vi "Measure distance.vi"(8 "error in (no error)":errorcluster, 11 "Input image":T3=refnum) -> (0 "error out":errorcluster)   [LabVIEW 2020]
uses:
  <vilib>/vision/Image Controls.llb/IMAQ Image.ctl
  <vilib>/vision/NI_Vision_Development_Module.lvlib
panel:
  in  "Clear Measurements":bool
  out "Distances":dbl[][](array[numeric])
  in  "Measurement Mode":T1(ring)
  in  "Re-instate":bool
  out "error out 11":errorcluster
  out "error out 10":errorcluster
  out "error out 9":errorcluster
  out "error out 8":errorcluster
  out "Distances":sgl[](array[numeric]) format="%.4f"
  out "output cluster":T2 {"Y" format="%.2f"; "X" format="%.2f"}
  out "min value":dbl
  out "Array 2":dbl[](array[numeric])
  out "Array":cdb[](array[numeric])
  out "Coordinates":i32[](array[numeric])
  out "Last Mouse Position:All Elements":cluster{"X":i32, "Y":i32}
  out "Image Pixels (I16) 2":i16[][](array[numeric])
  in  "Tab Control 2":enum32{"Grayscale", "Binary", "Intensity"}(tab)
  out "Output Image":T3(plugin-control)
  in  "Grid":bool
  in  "Grid Lines":u32=2 min=1 max=100 step=1
  out "Output Image 2":T3(plugin-control)
  out "Intensity Graph":i16[][](graph)
  out "Image Pixels (U8)":u8[][](array[numeric])
  out "error out 7":errorcluster
  out "Maximal Value":sgl
  out "Minimal Value":sgl
  in  "Number of iterations (1)":i32=1
  in  "Max Radius":sgl=100.0
  in  "Min Radius":sgl=3.0
  out "error out 6":errorcluster
  out "Circles Data":T4(array[cluster])
  in  "Operation":T5(ring)
  out "error out 5":errorcluster
  out "error out 4":errorcluster
  out "error out 3":errorcluster
  out "Image Pixels (I16)":i16[][](array[numeric])
  out "error out 2":errorcluster
  in  "Vertical Pointer Slide":cluster{"Numeric":dbl, "Numeric":dbl}(slide)={"Numeric"=0.0, "Numeric"=254.0} scale=0.0..4096.0
  in  "stop":bool
  # "X Start"
  # "Y start"
  # "X Stop"
  # "X Dist"
  # "Dist"
  # "Y Stop"
  # "Y Dist"
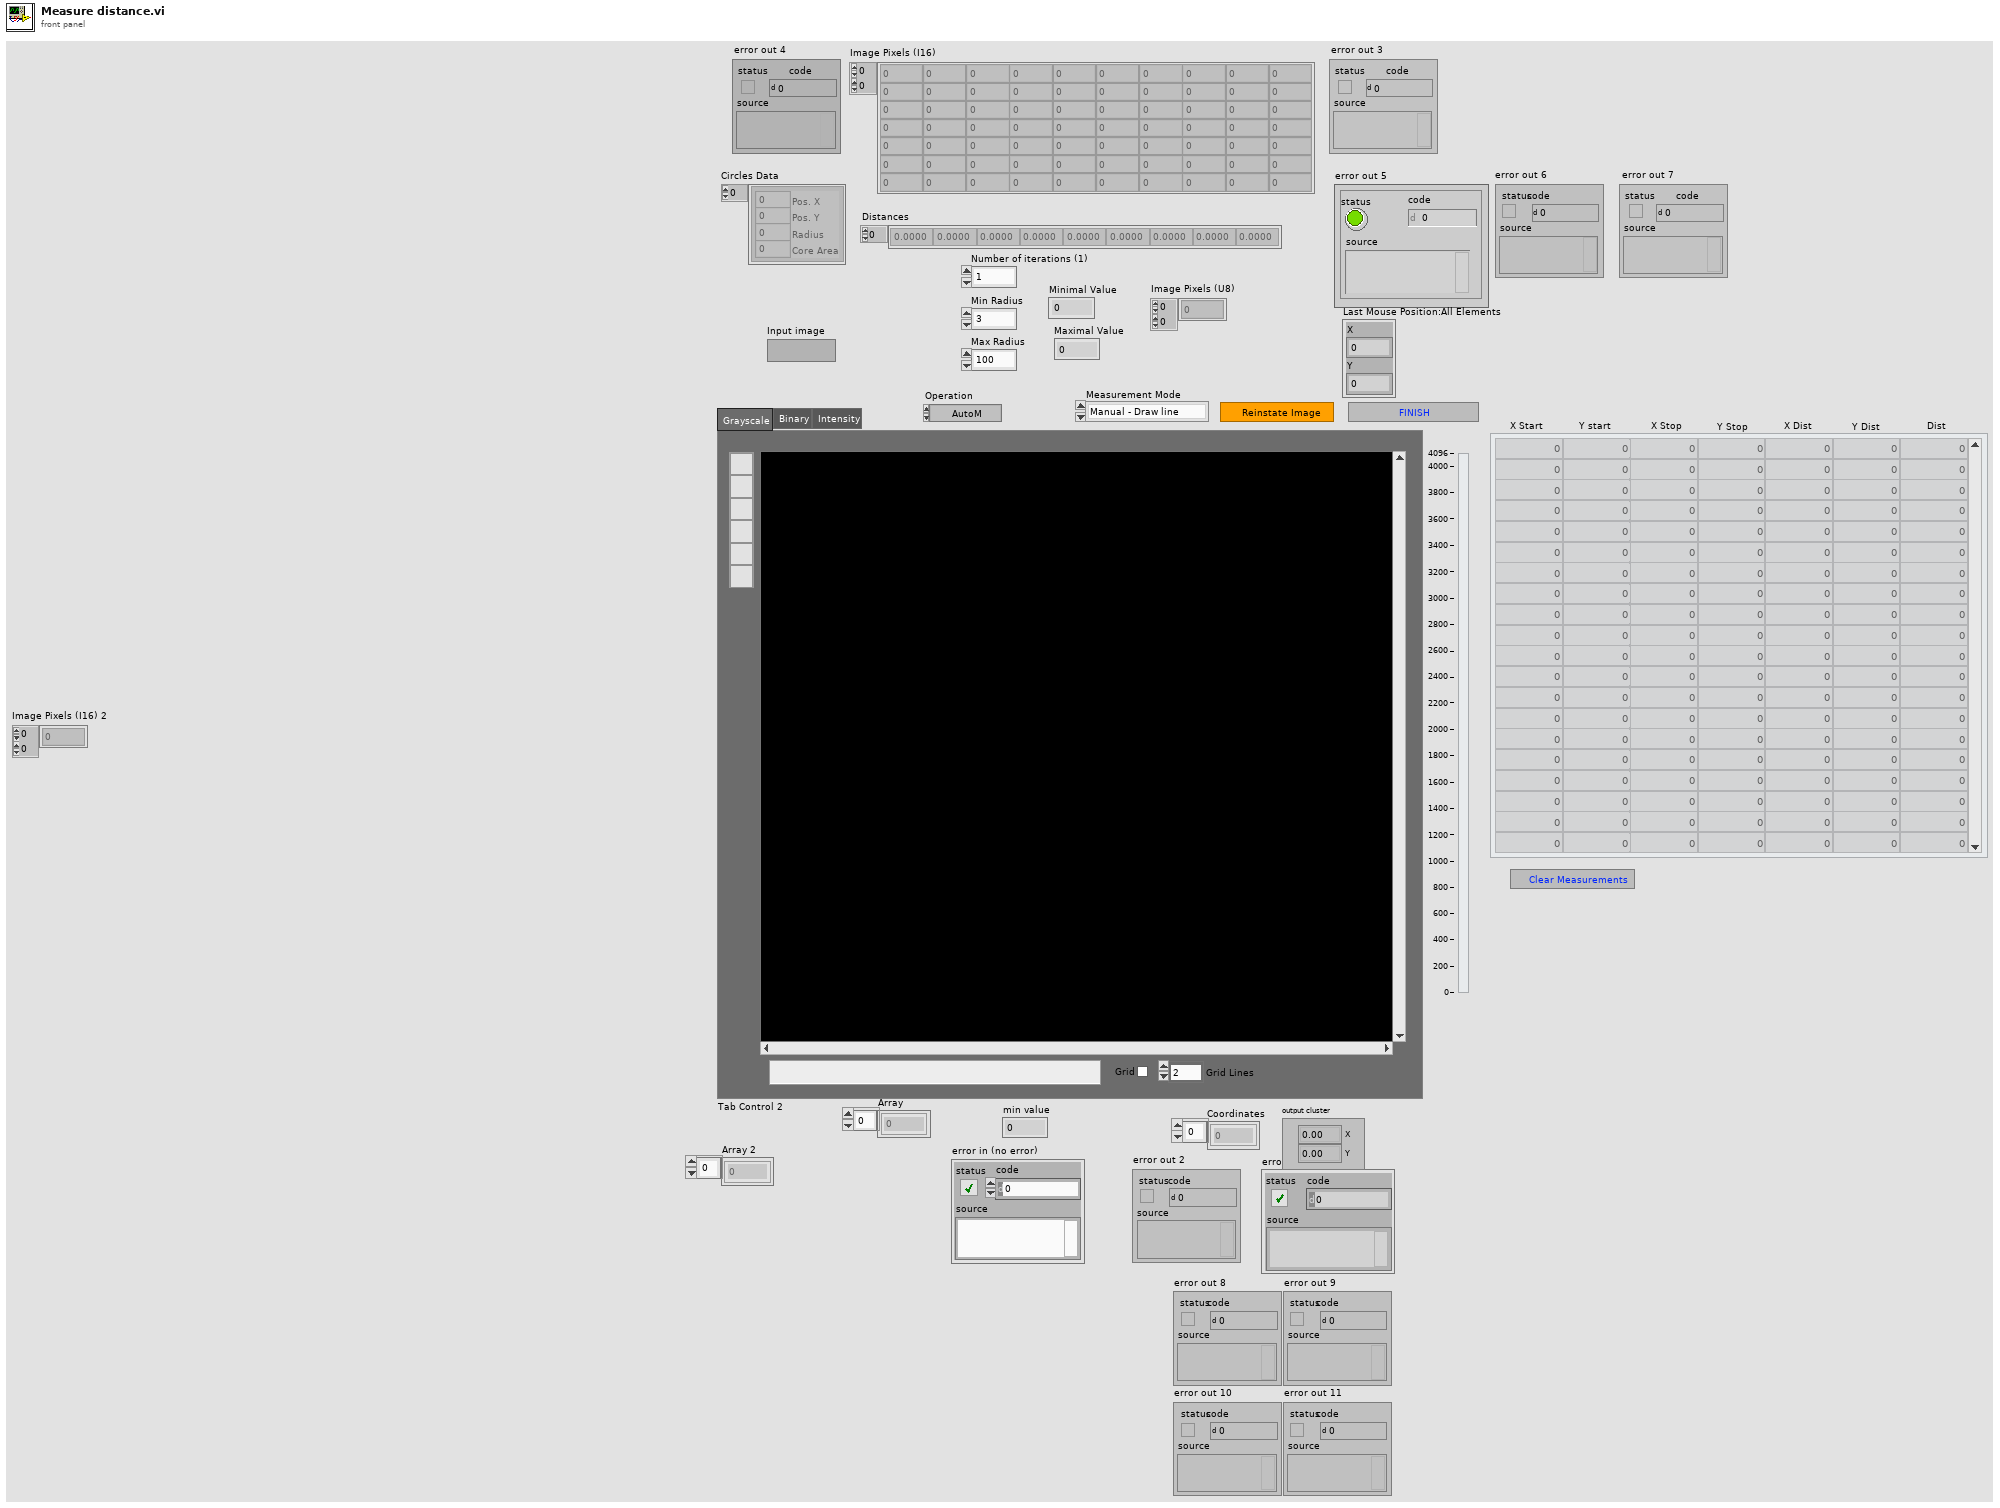
[diagram p1: front panel]
types:
  T1 = enum16{"Manual - Draw line", "Manual - Circles", "Manual - Points", "Automatic - Circles", "Automatic - Points"}
  T2 = typedef "IMAQ Point" = cluster{"X":sgl, "Y":sgl}
  T3 = typedef "IMAQ Image.ctl" = refnum<image>
  T4 = cluster{"Pos. X":i32, "Pos. Y":i32, "Radius":i32, "Core Area":i32}[]
  T5 = enum32{"AutoM", "Close", "Dilate", "Erode", "Gradient", "Gradient out", "Gradient in", "Hit miss", "Open", "PClose", "POpen", "Thick", "Thin"}
  T6 = typedef "ROI Descriptor" = cluster{"Global Rectangle":i32[], "Contours":cluster{"ID":enum32{"External", "Internal"}, "Type":u32, "Coordinates":i32[]}[]}
  T7 = typedef "IMAQ Circle" = cluster{"Center X":i32, "Center Y":i32, "Inner Radius":i32, "Outer Radius":i32, "Start Angle":dbl, "End Angle":dbl}
  T8 = typedef "Image Type" = u32
  T9 = cluster{"histogram":u32[], "Minimal Value":sgl, "Maximal Value":sgl, "Starting Value":sgl, "Interval Width":sgl, "Mean Value":sgl, "Standard  Variation":sgl, "Area (pixels)":i32}
  T10 = typedef "IMAQ Line" = cluster{"Start X":i32, "Start Y":i32, "End X":i32, "End Y":i32}
  T11 = cluster{"Pos. X":i32, "Pos. Y":i32, "Radius":i32, "Core Area":i32}
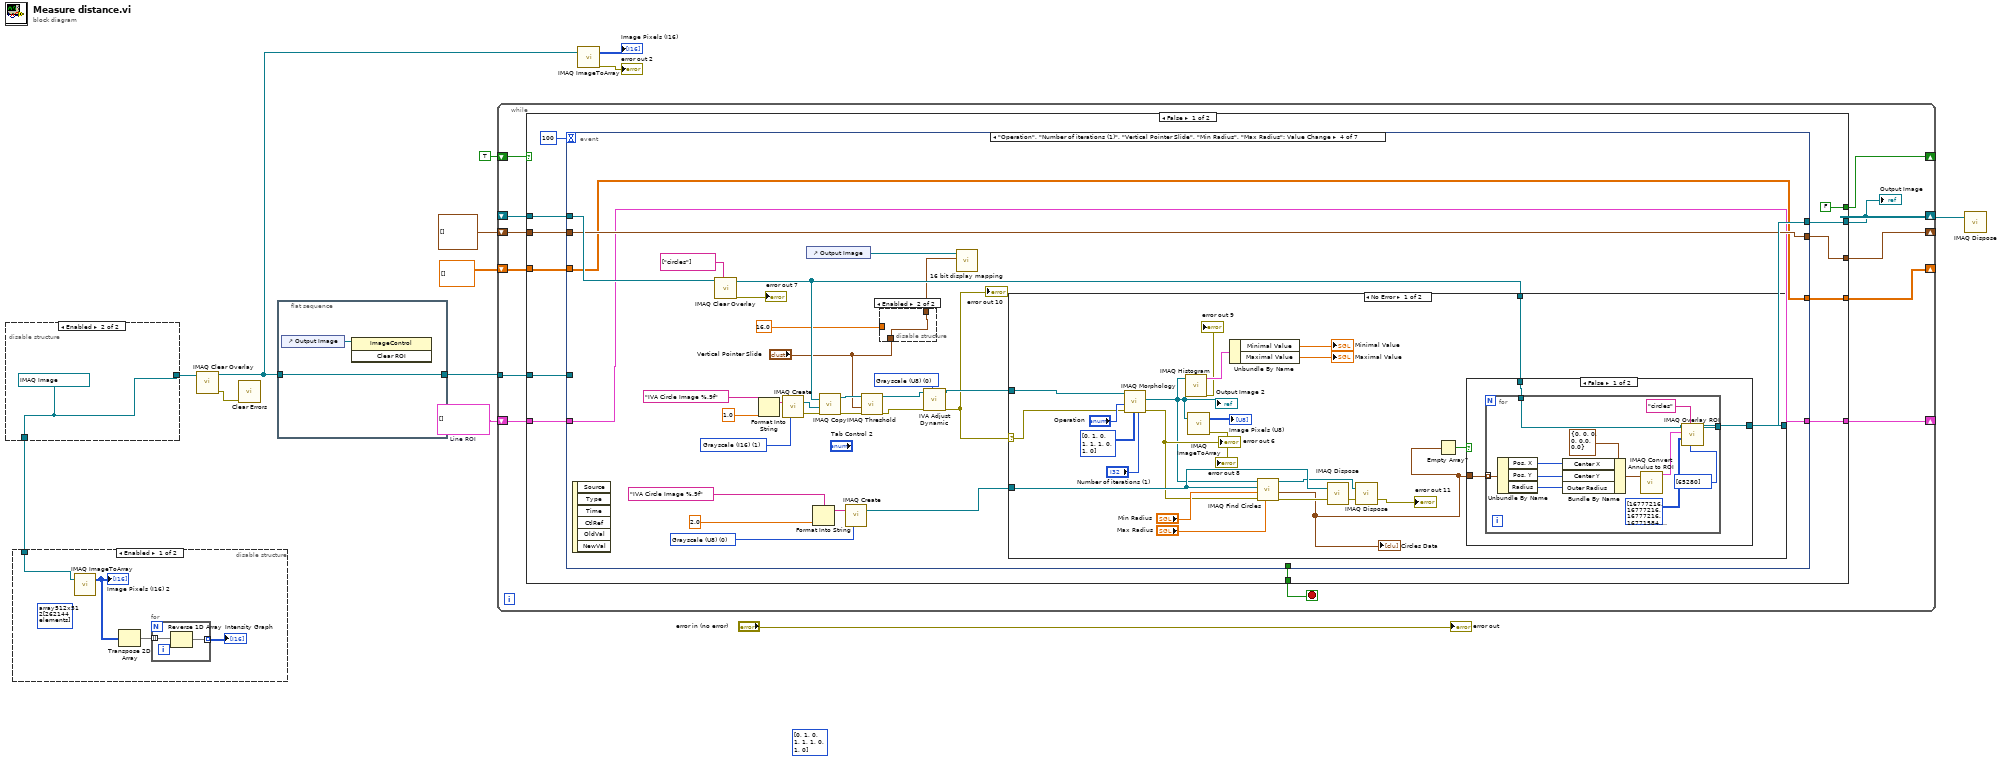
[diagram p0: block diagram]
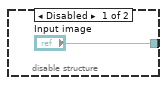
[diagram p2: hidden frame]
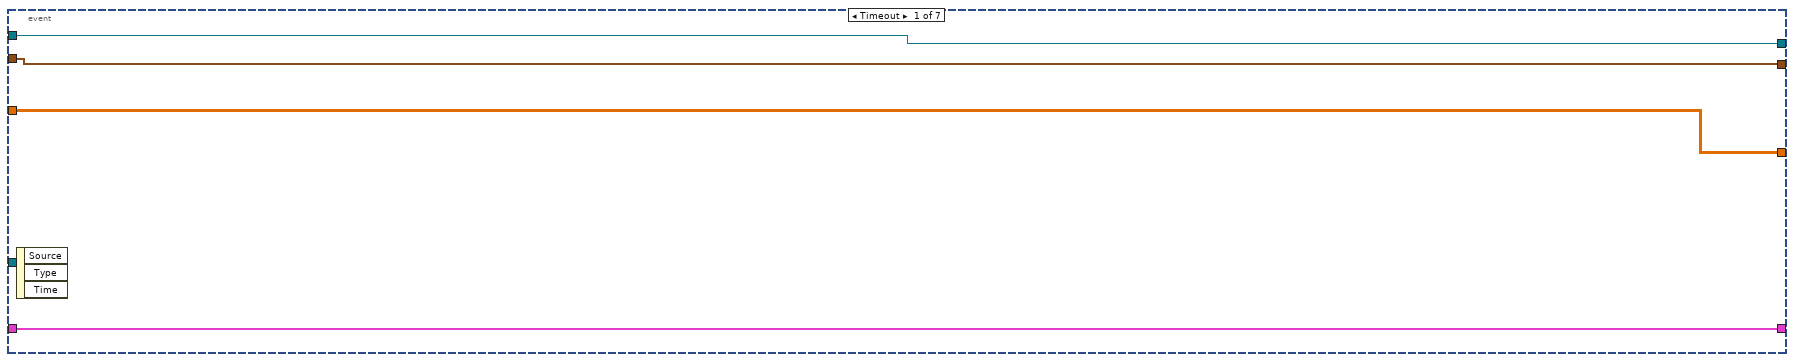
[diagram p4: hidden frame]
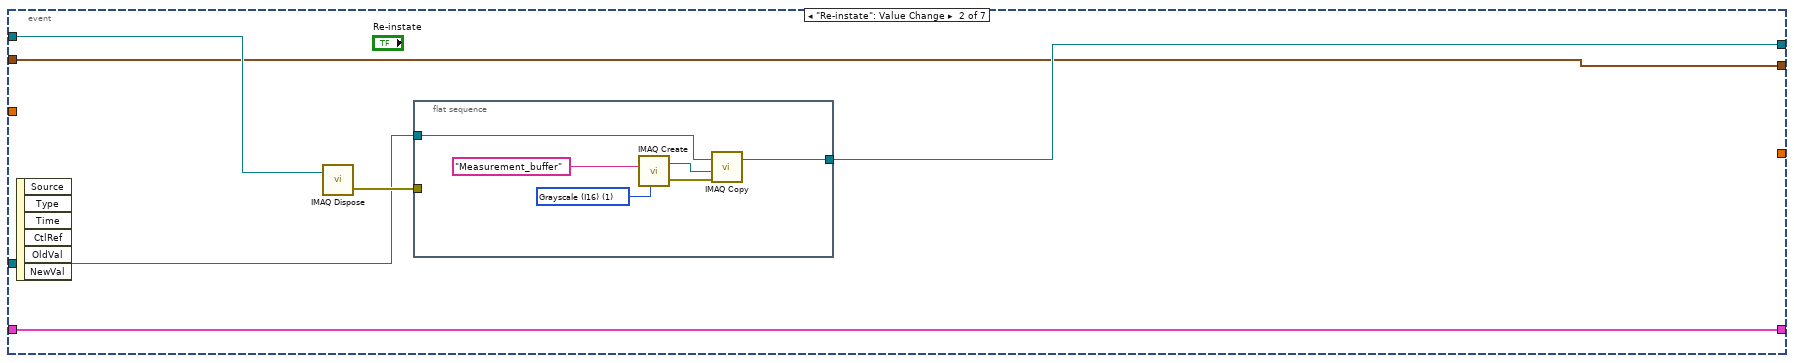
[diagram p5: hidden frame]
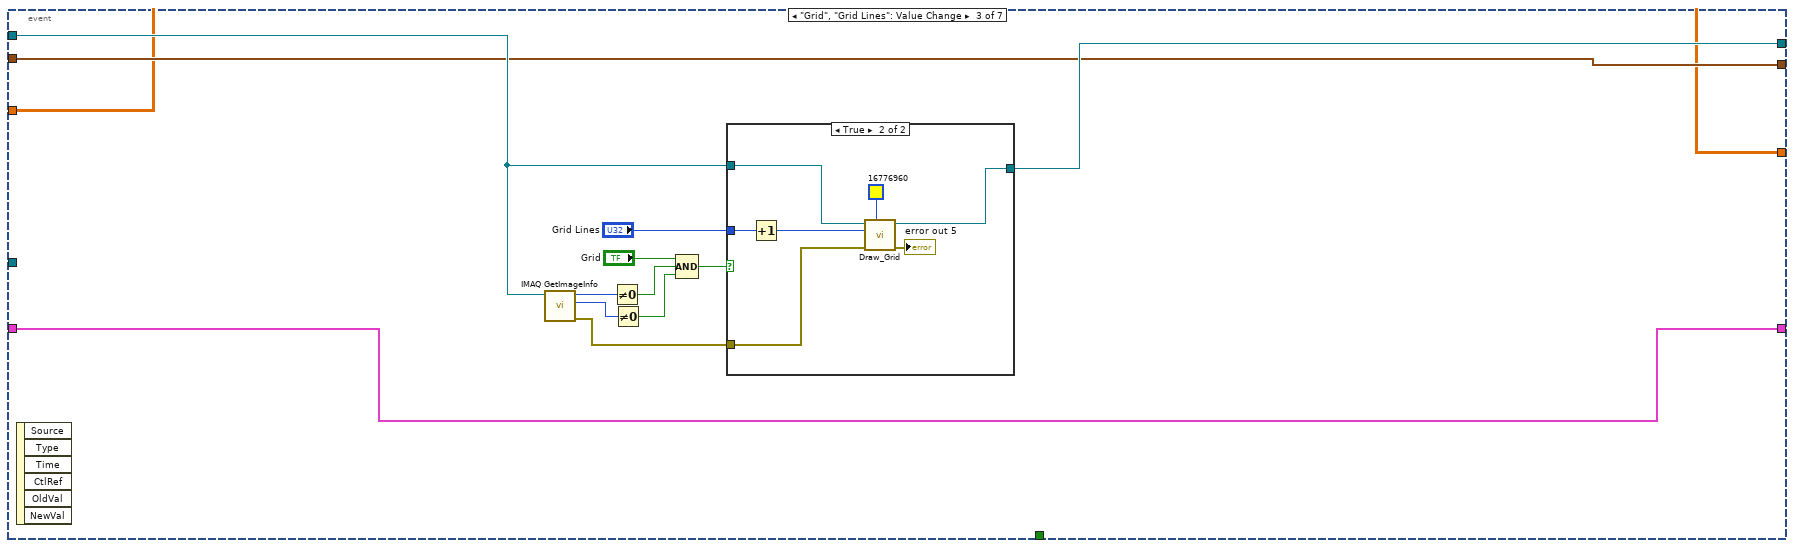
[diagram p6: hidden frame]
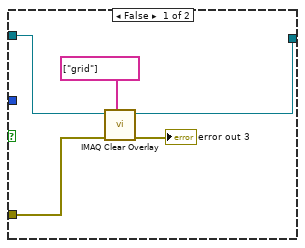
[diagram p7: hidden frame]
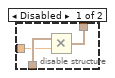
[diagram p8: hidden frame]
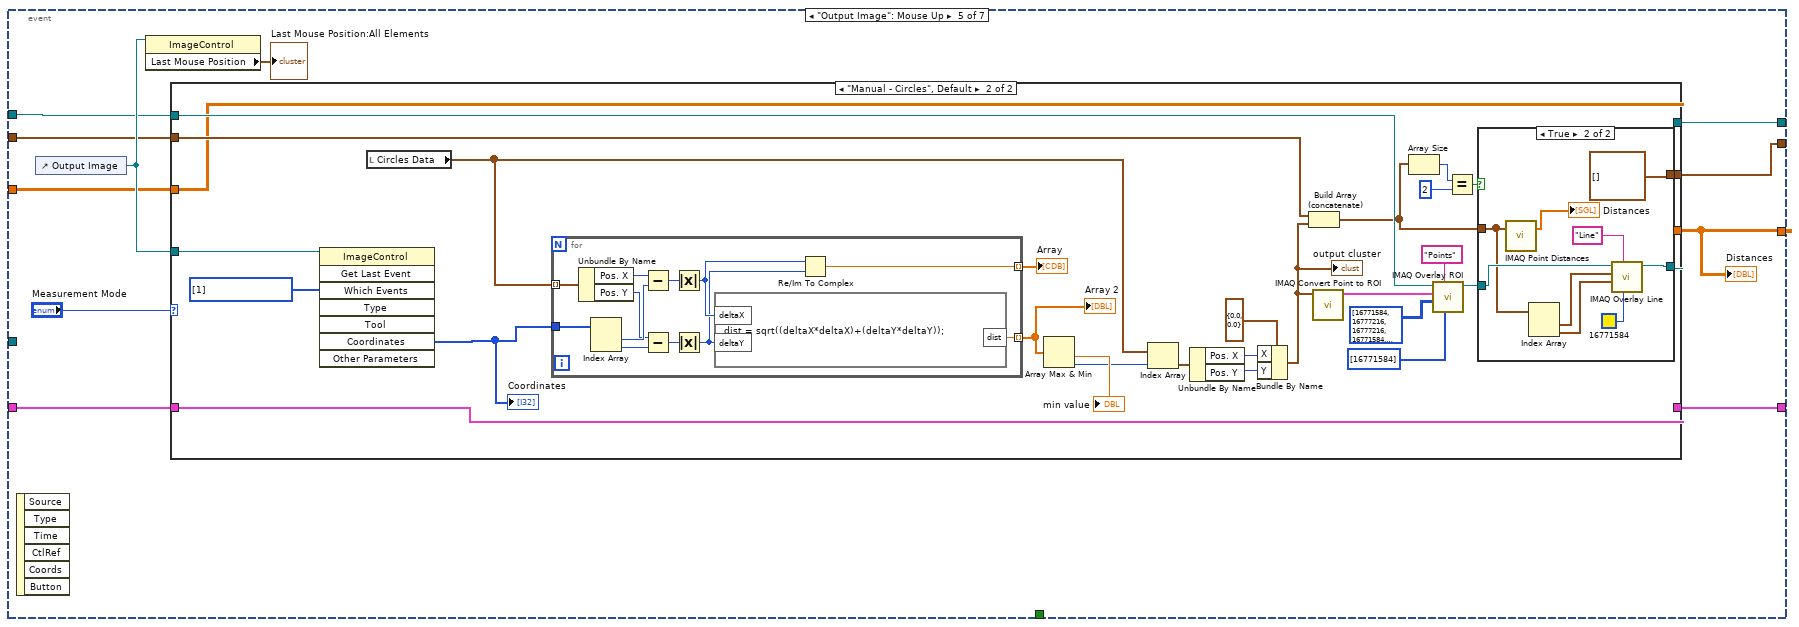
[diagram p11: hidden frame]
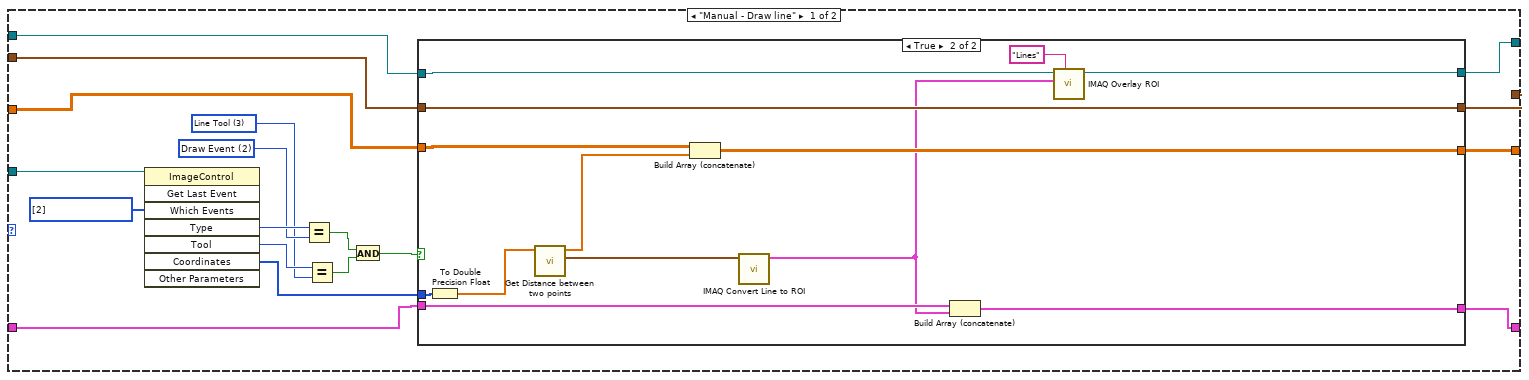
[diagram p12: hidden frame]
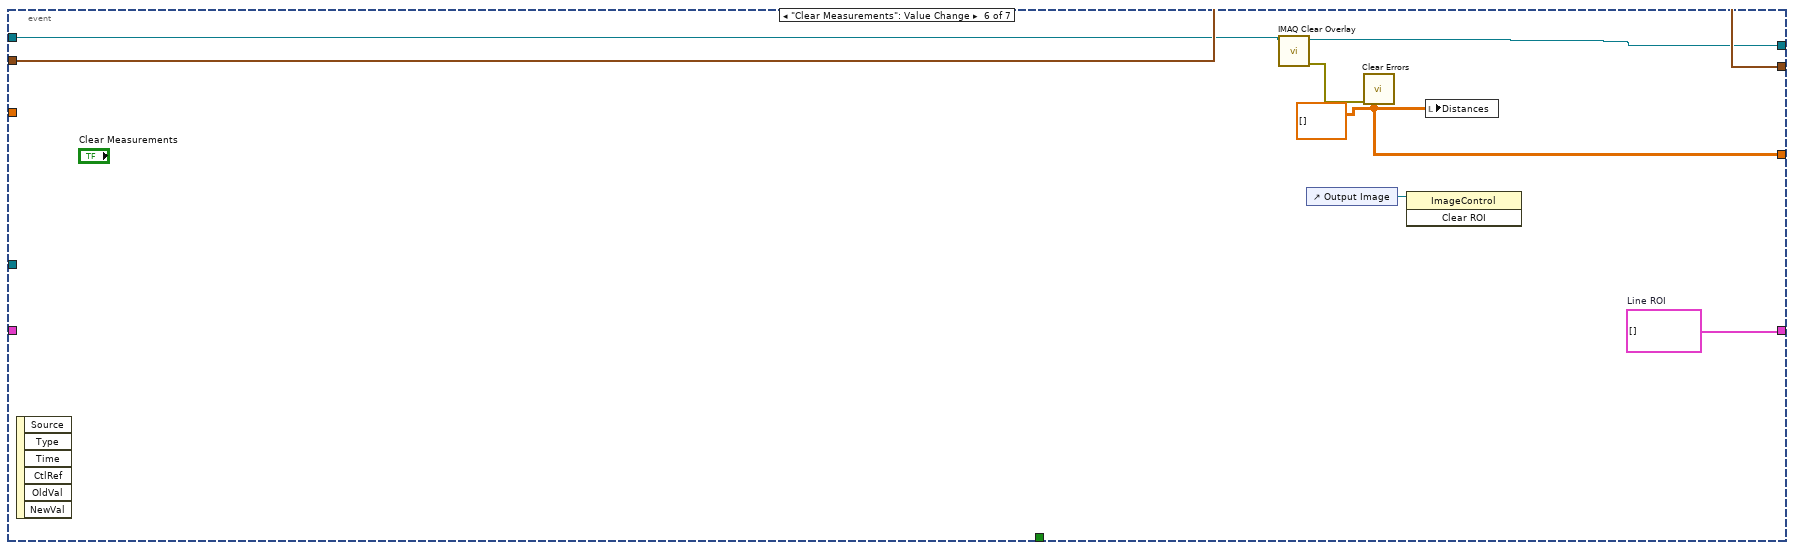
[diagram p15: hidden frame]
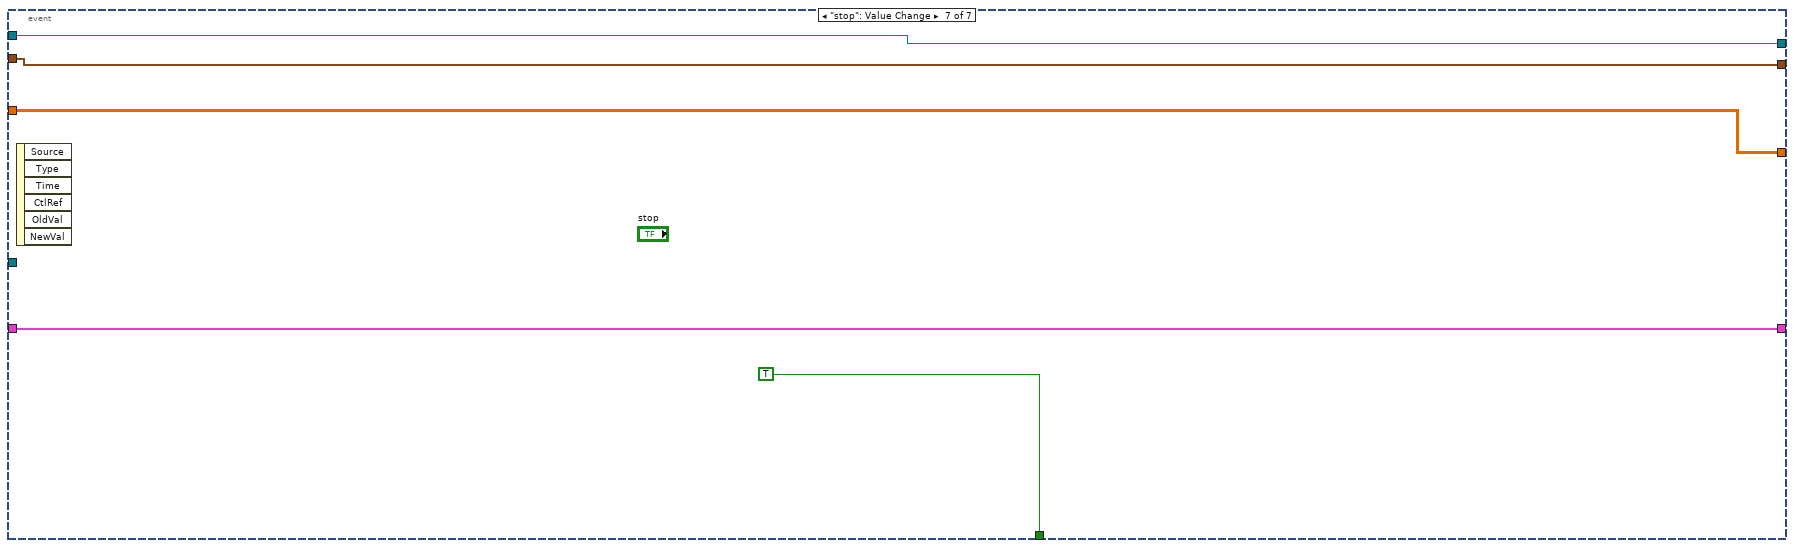
[diagram p16: hidden frame]
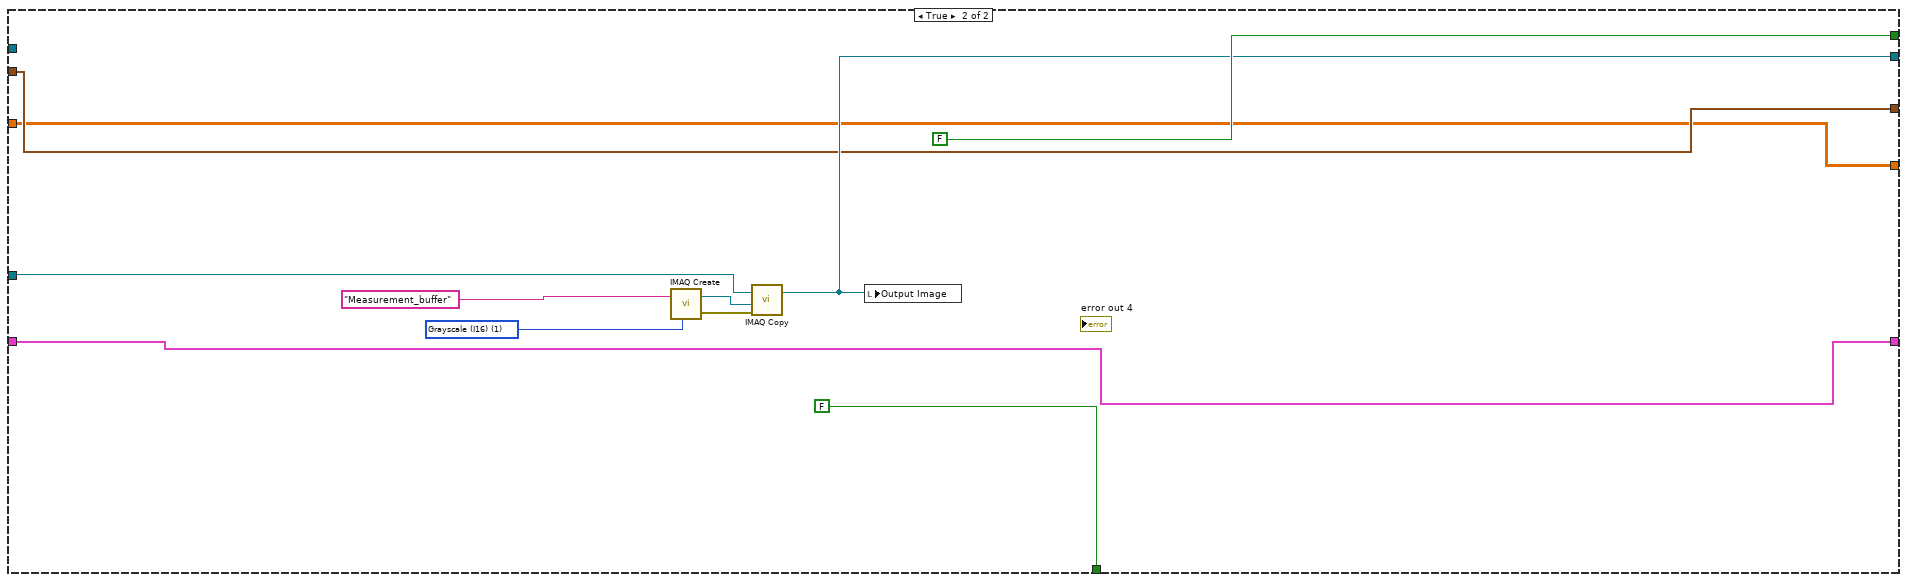
[diagram p17: hidden frame]
diagram:
  w5 = T6[] []  # Line ROI
  (unwired) i32[][] [[0, 1, 0], [1, 1, 1], [0, 1, 0]] ("Structuring Element (Basic Morphology 1) 2")
  n1 = disable-structure shown="Enabled" {
    disable-tunnel: ["Input image" w15] -> w4
    disable-tunnel: [_ w15] -> w8
    frame Disabled {
    }
    frame Enabled {
      w15 = T3 refnum ("Input image 2")
    }
  }
  n2 = disable-structure shown="Enabled" {
    disable-tunnel: w8 -> [w19 _]
    frame Enabled {
      (unwired) i16[][] array512x512[262144 elements] ("Image Pixels (I16) 2")
      n3 = call "IMAQ ImageToArray"("Image"=w19) -> ("Image Pixels (I16)"=w17:i16[][])  [unwired: 3 in, 4 out]
      "Image Pixels (I16) 2" <- w17
      n4 = Transpose 2D Array(2D array=w17) -> (transposed array=w18:i16[][])
      n5 = for {
        tunnel: w18 -> [w21] mode=indexing
        tunnel: [w20] -> w16 mode=indexing
        n6 = Reverse 1D Array(array=w21) -> (reversed array=w20:i16[])
      }
      "Intensity Graph" <- w16
    }
    frame Disabled {
    }
  }
  n7 = call "IMAQ Clear Overlay"("Image"=w4) -> ("error out"=w3:errorcluster, "Image Out"=w2:T3)  [unwired: 9 in]
  n8 = call <vilib>:"Clear Errors.vi"("error in (no error)"=w3) -> ()  [unwired: 5 in, 2 out]
  n9 = flat-sequence {
    tunnel: w2 -> [w23]
    tunnel: [w23] -> w1
    frame #0 {
      n10 = control-ref of="Output Image"() -> (w22:refnum<vi>)
      n11 = invoke class="ImageControl" method="Clear ROI"(reference=w22) -> ()  [unwired: 2 in, 3 out]
    }
  }
  n12 = while {
    shift-right: [w31] -> _
    shift-left: TRUE -> [w35]
    tunnel: w1 -> [w34]
    shift-right: [w30] -> w7
    shift-left: _ -> [w33]
    shift-right: [w28] -> _
    shift-left: T2[] [] -> [w29]
    shift-right: [w26] -> _
    shift-left: dbl[][] [] ("Distances 2") -> [w27]
    shift-right: [w24] -> _
    shift-left: w5 -> [w25]
    stop <- w32 stop-if-true
    n13 = case shown="False" w35 {
      tunnel: w34 -> [w40 w279]
      tunnel: [w46 w277] -> w30
      tunnel: w33 -> [w47 _]
      tunnel: [w44 FALSE] -> w32
      tunnel: [FALSE FALSE] -> w31
      tunnel: w29 -> [w42 w276]
      tunnel: [w41 w276] -> w28
      tunnel: w27 -> [w39 w274]
      tunnel: [w38 w274] -> w26
      tunnel: w25 -> [w37 w273]
      tunnel: [w36 w273] -> w24
      frame False {
        n14 = event shown="[3] \"Operation\", \"Number of iterations (1)\", \"Vertical Pointer Slide\", \"Min Radius\", \"Max Radius\": Value Change" {
          selector: _ -> [_ _ _ _ _ _ _]
          dyn-events: _ -> [_ _ _ _ _ _ _]
          timeout: 100 -> [_ _ _ _ _ _ _]
          tunnel: w47 -> [w51 w57 w75 w104 w172 w264 w271]
          tunnel: [w51 w54 w76 w106 w171 w262 w271] -> w46
          tunnel: [_ _ _ _ _ _ TRUE] -> w44
          tunnel: w42 -> [w50 w53 w66 w101 w169 w265 w270]
          tunnel: [w50 w53 w66 w101 w170 w265 w270] -> w41
          tunnel: w40 -> [_ w55 _ _ _ _ _]
          tunnel: w39 -> [w49 _ w65 w97 w167 _ w269]
          tunnel: [w49 _ w65 w97 w164 w267 w269] -> w38
          tunnel: w37 -> [w48 w52 w64 w96 w166 _ w268]
          tunnel: [w48 w52 w64 w96 w165 w266 w268] -> w36
          event Timeout {
            n15 = event-data() -> ()  [unwired: 1 in, 3 out]
          }
          event "Re-instate": Value Change {
            n16 = event-data() -> ()  [unwired: 1 in, 6 out]
            n17 = call "IMAQ Dispose"("Image"=w57) -> ("error out"=w56:errorcluster)  [unwired: 5 in]
            n18 = flat-sequence {
              tunnel: w56 -> [_]
              tunnel: w55 -> [w59]
              tunnel: [w58] -> w54
              frame #0 {
                w60 = T8 1 items=["Grayscale (U8)", "Grayscale (I16)", "Grayscale (SGL)", "Complex (CSG)", "RGB (U32)", "HSL (U32)", "RGB (U64)", "Grayscale (U16)"] ("Image Type")
                n19 = call "IMAQ Create"("Image Name"="Measurement_buffer", "Image Type"=w60) -> ("New Image"=w62:T3, "error out"=w63:errorcluster)  [unwired: 3 in]
                n20 = call "IMAQ Copy"("error in (no error)"=w63, "Image Dst"=w62, "Image Src"=w59) -> ("Image Dst Out"=w58:T3)  [unwired: 3 in, 1 out]
              }
            }
          }
          event "Grid", "Grid Lines": Value Change {
            n21 = event-data() -> ()  [unwired: 1 in, 6 out]
            n22 = call "IMAQ GetImageInfo"("Image"=w75) -> ("error out"=w69:errorcluster, "Y Resolution"=w72:i32, "X Resolution"=w73:i32)  [unwired: 3 in, 5 out]
            n23 = Not Equal To 0?(x=w73) -> (x != 0?=w71:bool)
            n24 = Not Equal To 0?(x=w72) -> (x != 0?=w70:bool)
            n25 = Compound Arithmetic op=AND("Grid", w71, w70) -> (w68:bool)
            n26 = case shown="True" w68 {
              tunnel: w75 -> [w80 w88]
              tunnel: [w79 w87] -> w76
              tunnel: w69 -> [w77 w85]
              tunnel: "Grid Lines" -> [_ w83]
              frame False {
                n27 = call "IMAQ Clear Overlay"("Groups"=string[] ["grid"], "error in (no error)"=w77, "Image"=w80) -> ("error out"=→"error out 3":errorcluster, "Image Out"=w79:T3)  [unwired: 7 in]
              }
              frame True {
                n28 = Increment(x=w83) -> (x+1=w82:u32)
                n29 = call "Draw_Grid.vi"("Grid Line Color"=u32 16776960, "error in (no error)"=w85, "Grid Lines"=w82, "Image In"=w88) -> ("error out"=→"error out 5":errorcluster, "Image Out"=w87:T3)  [unwired: 6 in]
              }
            }
          }
          event "Operation", "Number of iterations (1)", "Vertical Pointer Slide", "Min Radius", "Max Radius": Value Change {
            w110 = T8 0 items=["Grayscale (U8)", "Grayscale (I16)", "Grayscale (SGL)", "Complex (CSG)", "RGB (U32)", "HSL (U32)", "RGB (U64)", "Grayscale (U16)"] ("Image Type")
            w111 = T8 0 items=["Grayscale (U8)", "Grayscale (I16)", "Grayscale (SGL)", "Complex (CSG)", "RGB (U32)", "HSL (U32)", "RGB (U64)", "Grayscale (U16)"] ("Image Type")
            w116 = T8 1 items=["Grayscale (U8)", "Grayscale (I16)", "Grayscale (SGL)", "Complex (CSG)", "RGB (U32)", "HSL (U32)", "RGB (U64)", "Grayscale (U16)"] ("Image Type")
            n30 = event-data() -> ()  [unwired: 1 in, 6 out]
            n31 = call "IMAQ Clear Overlay"("Groups"=string[] ["circles"], "Image"=w104) -> ("error out"=→"error out 7":errorcluster, "Image Out"=w103:T3)  [unwired: 8 in]
            n32 = Format Into String(format string="IVA Circle Image %.9f" ("Image Name"), 1.0) -> (resulting string=w118:string)  [unwired: 2 in, 1 out]
            n33 = call "IMAQ Create"("Image Name"=w118, "Image Type"=w116) -> ("New Image"=w108:T3, "error out"=w109:errorcluster)  [unwired: 2 in, 1 out]
            n34 = control-ref of="Output Image"() -> (w100:refnum<vi>)
            n35 = Format Into String(format string="IVA Circle Image %.9f" ("Image Name"), 2.0) -> (resulting string=w114:string)  [unwired: 2 in, 1 out]
            n36 = call "IMAQ Copy"("error in (no error)"=w109, "Image Dst"=w108, "Image Src"=w103) -> ("error out"=w94:errorcluster, "Image Dst Out"=w95:T3)  [unwired: 3 in]
            n37 = call "IMAQ Create"("Image Name"=w114, "Image Type"=w111) -> ("New Image"=w107:T3)  [unwired: 2 in, 2 out]
            n38 = call "IMAQ Threshold"("error in (no error)"=w94, "Range"="Vertical Pointer Slide", "Image Src"=w95) -> ("error out"=w93:errorcluster, "Image Dst Out"=w92:T3)  [unwired: 3 in, 4 out]
            n39 = disable-structure shown="Enabled" {
              disable-tunnel: "Vertical Pointer Slide" -> [w121 w122]
              disable-tunnel: 16.0 -> [w120 _]
              disable-tunnel: [w119 w122] -> w98
              frame Disabled {
                n40 = Multiply(x=w121, y=w120) -> (x*y=w119:cluster{"Numeric":dbl, "Numeric":dbl})
              }
              frame Enabled {
              }
            }
            n41 = call <vilib>:"IVA Adjust Dynamic.vi"("Image Type"=w110, "error in (no error)"=w93, "Image Src"=w92) -> ("error out"=w90:errorcluster, "Image Out"=w91:T3)  [unwired: 7 out]
            "error out 10" <- w90
            n42 = call "16 bit display mapping.vi"("16 bit display mapping"=w98, "Image Display"=w100) -> ()  [unwired: 8 in, 2 out]
            n43 = case shown="No Error" w90 {
              selector: w90 -> [w123 _]
              tunnel: w107 -> [w141 w163]
              tunnel: [w138 w163] -> w106
              tunnel: w91 -> [w124 _]
              tunnel: w103 -> [w136 _]
              frame No Error {
                n44 = call "IMAQ Morphology"("Number of iterations (1)"="Number of iterations (1)", "Structuring Element"=i32[][] [[0, 1, 0], [1, 1, 1], [0, 1, 0]] ("Structuring Element (Basic Morphology 1) 2"), "error in (no error)"=w123, "Operation"="Operation", "Image Src"=w124) -> ("error out"=w132:errorcluster, "Image Dst Out"=w130:T3)  [unwired: 2 in, 3 out]
                "error out 6" <- w132
                "Output Image 2" <- w130
                n45 = call "IMAQ Histogram"("Image"=w130) -> ("error out"=→"error out 9":errorcluster, "Histogram Report"=w135:T9)  [unwired: 4 in, 5 out]
                n46 = call "IMAQ ImageToArray"("Image"=w130) -> ("error out"=→"error out 8":errorcluster, "Image Pixels (U8)"=→"Image Pixels (U8)":u8[][])  [unwired: 3 in, 3 out]
                n47 = Unbundle By Name(w135) -> ("Minimal Value"=→"Minimal Value":sgl, "Maximal Value"=→"Maximal Value":sgl)
                n48 = call "IMAQ Find Circles"("Max Radius"="Max Radius", "error in (no error)"=w132, "Min Radius"="Min Radius", "Image Dst"=w141, "Image Src"=w130) -> ("error out"=w142:errorcluster, "Circles Data"=w126:T4, "Image Dst Out"=w139:T3)  [unwired: 4 out]
                "Circles Data" <- w126
                n49 = call "IMAQ Dispose"("Image"=w141, "error in (no error)"=w142) -> ("error out"=w140:errorcluster)  [unwired: 1 in, 3 out]
                n50 = call "IMAQ Dispose"("Image"=w139, "error in (no error)"=w140) -> ("error out"=→"error out 11":errorcluster)  [unwired: 1 in, 3 out]
                n51 = Empty Array?(array=w126) -> (empty?=w125:bool)
                n52 = case shown="False" w125 {
                  tunnel: [w149 w162] -> w138
                  tunnel: w136 -> [w148 w162]
                  tunnel: w126 -> [w147 _]
                  frame False {
                    n53 = for {
                      tunnel: w147 -> [w160] mode=indexing
                      tunnel: w148 -> [w155]
                      tunnel: [w151] -> w149
                      n54 = Unbundle By Name(w160) -> ("Pos. X"=w159:i32, "Pos. Y"=w158:i32, "Radius"=w157:i32)
                      n55 = Bundle By Name(cluster=T7 {"Center X"=0, "Center Y"=0, "Inner Radius"=0, "Outer Radius"=0, "Start Angle"=0.0, "End Angle"=0.0} ("Annulus"), "Center X"=w159, "Center Y"=w158, "Outer Radius"=w157) -> (w156:T7)
                      n56 = call "IMAQ Convert Annulus to ROI"("Annulus"=w156) -> ("ROI Descriptor"=w154:T6)  [unwired: 8 in, 1 out]
                      n57 = call "IMAQ Overlay ROI"("Colors (Green)"=u32[] [65280], "Group"="circles", "Point Symbol"=u32[][] [[16777216, 16777216, 16777216, 16771584, 16777216, 16777216, 16777216], [16777216, 16777216, 16777216, 16771584, 16777216, 16777216, 16777216], [16777216, 16777216, 16777216, 16771584, 16777216, 16777216, 16777216], [16771584, 16771584, 16771584, 16771584, 16771584, 16771584, 16771584], [16777216, 16777216, 16777216, 16771584, 16777216, 16777216, 16777216], [16777216, 16777216, 16777216, 16771584, 16777216, 16777216, 16777216], [16777216, 16777216, 16777216, 16771584, 16777216, 16777216, 16777216]], "ROI Descriptor"=w154, "Image"=w155) -> ("Image Out"=w151:T3)  [unwired: 5 in, 1 out]
                    }
                  }
                  frame True {
                  }
                }
              }
              frame Error {
              }
            }
          }
          event "Output Image": Mouse Up {
            n58 = event-data() -> ()  [unwired: 1 in, 6 out]
            n59 = control-ref of="Output Image"() -> (w173:refnum<vi>)
            n60 = property class="ImageControl"(reference=w173) -> ("Last Mouse Position"=→"Last Mouse Position:All Elements":cluster{"X":i32, "Y":i32})  [unwired: 1 in, 2 out]
            n61 = case shown="\"Manual - Circles\", Default" "Measurement Mode" {
              tunnel: w173 -> [w191 w237]
              tunnel: w172 -> [w180 w223]
              tunnel: [w179 w217] -> w171
              tunnel: [w178 w216] -> w170
              tunnel: w169 -> [w177 w215]
              tunnel: w167 -> [w182 w211]
              tunnel: [w181 w211] -> w164
              tunnel: w166 -> [w176 w210]
              tunnel: [w175 w210] -> w165
              frame "Manual - Draw line" {
                w187 = 3 items=["None", "Selection Tool", "Point Tool", "Line Tool", "Rectangle Tool", "Oval Tool", "Polygon Tool", "ClosedFreehandTool", "Annulus Tool", "Rotated Rectangle Tool", "Zoom Tool", "Pan Tool", "Polyline Tool", "Freehand Tool"] ("Tool")
                w189 = 2 items=["No Event"=0, "Click Event"=1, "Draw Event"=2, "Size Event"=4, "Scroll Event"=5, "Double Click Event"=8] ("Type 2")
                w192 = i32[] [2] items=["No Event"=0, "Click Event"=1, "Draw Event"=2, "Size Event"=4, "Scroll Event"=5, "Double Click Event"=8] ("Which Events")
                n62 = invoke class="ImageControl" method="Get Last Event"(reference=w191, "Which Events"=w192) -> ("Type"=w190:i32, "Tool"=w188:i32, "Coordinates"=w183:i32[])  [unwired: 6 in, 5 out]
                n63 = Equal?(x=w190, y=w189) -> (x = y?=w186:bool)
                n64 = Equal?(x=w188, y=w187) -> (x = y?=w185:bool)
                n65 = And(x=w186, y=w185) -> (x .and. y?=w184:bool)
                n66 = case shown="True" w184 {
                  tunnel: w183 -> [_ w209]
                  tunnel: w182 -> [w196 w207]
                  tunnel: [w196 w206] -> w181
                  tunnel: w180 -> [w195 w204]
                  tunnel: [w195 w203] -> w179
                  tunnel: [w194 w202] -> w178
                  tunnel: w177 -> [w194 w202]
                  tunnel: w176 -> [w193 w201]
                  tunnel: [w193 w200] -> w175
                  frame False {
                  }
                  frame True {
                    n67 = To Double Precision Float(number=w209) -> (double precision float=w208:dbl[])
                    n68 = call "Get Distance between two points.vi"("Array"=w208) -> ("Line ROI coordinates"=w197:T10, "appended array"=w205:dbl[])  [unwired: 9 in]
                    n69 = Build Array (concatenate)(w207, w205) -> (w206:dbl[][])
                    n70 = call "IMAQ Convert Line to ROI"("Line"=w197) -> ("ROI Descriptor"=w199:T6)  [unwired: 8 in, 1 out]
                    n71 = Build Array (concatenate)(w201, w199) -> (w200:T6[])
                    n72 = call "IMAQ Overlay ROI"("Group"="Lines", "ROI Descriptor"=w199, "Image"=w204) -> ("Image Out"=w203:T3)  [unwired: 7 in, 1 out]
                  }
                }
              }
              frame "Manual - Circles", Default {
                w212 = i32[] [1] items=["No Event"=0, "Click Event"=1, "Draw Event"=2, "Size Event"=4, "Scroll Event"=5, "Double Click Event"=8] ("Which Events")
                n73 = invoke class="ImageControl" method="Get Last Event"(reference=w237, "Which Events"=w212) -> ("Coordinates"=w233:i32[])  [unwired: 6 in, 7 out]
                "Coordinates" <- w233
                n74 = local read "Circles Data"() -> (w224:T4)
                n75 = for {
                  tunnel: w224 -> [w260] mode=indexing
                  tunnel: w233 -> [w259]
                  tunnel: [w254] -> w235 mode=indexing
                  tunnel: [w253] -> w236 mode=indexing
                  n76 = Unbundle By Name(w260) -> ("Pos. X"=w252:i32, "Pos. Y"=w250:i32)
                  n77 = Index Array(array=w259) -> (element #1=w251:i32, element #2=w249:i32)  [unwired: 2 in]
                  n78 = Subtract(x=w252, y=w251) -> (x-y=w258:i32)
                  n79 = Subtract(x=w250, y=w249) -> (x-y=w257:i32)
                  n80 = Absolute Value(x=w258) -> (abs(x)=w256:i32)
                  n81 = Absolute Value(x=w257) -> (abs(x)=w255:i32)
                  n82 = formula code="dist = sqrt((deltaX*deltaX)+(deltaY*deltaY));"("deltaX"=w256, "deltaY"=w255) -> ("dist"=w254:dbl)
                  n83 = Re/Im To Complex(1:w255, 2:w256) -> (0:w253:cdb)
                }
                "Array" <- w236
                "Array 2" <- w235
                n84 = Array Max & Min(array=w235) -> (min value=→"min value":dbl, min index (indices)=w222:i32)  [unwired: 2 out]
                n85 = Index Array(array=w224, index=w222) -> (element=w232:T11)
                n86 = Unbundle By Name(w232) -> ("Pos. X"=w231:i32, "Pos. Y"=w230:i32)
                n87 = Bundle By Name(cluster=T2 {"X"=0.0, "Y"=0.0} ("Point"), "X"=w231, "Y"=w230) -> (w214:T2)
                "output cluster" <- w214
                n88 = Build Array (concatenate)(w215, w214) -> (w213:T2[])
                n89 = call "IMAQ Convert Point to ROI"("Point"=w214) -> ("ROI Descriptor"=w228:T6)  [unwired: 8 in, 1 out]
                n90 = Array Size(array=w213) -> (size(s)=w221:i32)
                n91 = call "IMAQ Overlay ROI"("Colors (Green)"=u32[] [16771584], "Group"="Points", "Point Symbol"=u32[][] [[16771584, 16777216, 16777216, 16771584, 16777216, 16777216, 16771584], [16777216, 16771584, 16777216, 16771584, 16777216, 16771584, 16777216], [16777216, 16777216, 16771584, 16771584, 16771584, 16777216, 16777216], [16771584, 16771584, 16771584, 16771584, 16771584, 16771584, 16771584], [16777216, 16777216, 16771584, 16771584, 16771584, 16777216, 16777216], [16777216, 16771584, 16777216, 16771584, 16777216, 16771584, 16777216], [16771584, 16777216, 16777216, 16771584, 16777216, 16777216, 16771584]], "ROI Descriptor"=w228, "Image"=w223) -> ("Image Out"=w218:T3)  [unwired: 5 in, 1 out]
                n92 = Equal?(x=w221, y=2) -> (x = y?=w219:bool)
                n93 = case shown="True" w219 {
                  tunnel: w213 -> [w238 w244]
                  tunnel: w218 -> [w239 w247]
                  tunnel: [w239 w246] -> w217
                  tunnel: [w238 T2[] []] -> w216
                  frame False {
                  }
                  frame True {
                    n94 = call "IMAQ Point Distances"("Points"=w244) -> ("Distances"=→"Distances":sgl[])  [unwired: 4 in, 1 out]
                    n95 = Index Array(array=w244) -> (element #1=w243:T2, element #2=w242:T2)  [unwired: 2 in]
                    n96 = call "IMAQ Overlay Line"("Color"=u32 16771584, "Group"="Line", "End Point"=w242, "Start Point"=w243, "Image"=w247) -> ("Image Out"=w246:T3)  [unwired: 5 in, 1 out]
                  }
                }
              }
            }
            "Distances" <- w164
          }
          event "Clear Measurements": Value Change {
            w266 = T6[] []  # Line ROI
            w267 = dbl[][] [] ("Distances 2")
            n97 = event-data() -> ()  [unwired: 1 in, 6 out]
            n98 = call "IMAQ Clear Overlay"("Image"=w264) -> ("error out"=w263:errorcluster, "Image Out"=w262:T3)  [unwired: 9 in]
            n99 = control-ref of="Output Image"() -> (w261:refnum<vi>)
            n100 = call <vilib>:"Clear Errors.vi"("error in (no error)"=w263) -> ()  [unwired: 5 in, 2 out]
            n101 = invoke class="ImageControl" method="Clear ROI"(reference=w261) -> ()  [unwired: 2 in, 3 out]
            n102 = local write "Distances"(w267) -> ()
          }
          event "stop": Value Change {
            n103 = event-data() -> ()  [unwired: 1 in, 6 out]
          }
        }
      }
      frame True {
        w283 = T8 1 items=["Grayscale (U8)", "Grayscale (I16)", "Grayscale (SGL)", "Complex (CSG)", "RGB (U32)", "HSL (U32)", "RGB (U64)", "Grayscale (U16)"] ("Image Type")
        n104 = call "IMAQ Create"("Image Name"="Measurement_buffer", "Image Type"=w283) -> ("New Image"=w278:T3, "error out"=w282:errorcluster)  [unwired: 3 in]
        n105 = call "IMAQ Copy"("error in (no error)"=w282, "Image Dst"=w278, "Image Src"=w279) -> ("Image Dst Out"=w277:T3)  [unwired: 3 in, 1 out]
        n106 = local write "Output Image"(w277) -> ()
      }
    }
    "Output Image" <- w30
  }
  n107 = call "IMAQ ImageToArray"("Image"=w2) -> ("error out"=→"error out 2":errorcluster, "Image Pixels (I16)"=→"Image Pixels (I16)":i16[][])  [unwired: 3 in, 3 out]
  n108 = call "IMAQ Dispose"("Image"=w7) -> ()  [unwired: 5 in, 1 out]
  "error out" <- "error in (no error)"
